vi "Down Sample Data.vi"(7 "Data log":enum16{"1 Hz", "10 Hz"}(ring), 8 "error in (no error)":errorcluster, 11 "location":path) -> (0 "error out":errorcluster)   [LabVIEW 2018]
uses:
  <vilib>/Analysis/baseanly.llb/Mean (DBL).vi
  <vilib>/Utility/file.llb/Read Delimited Spreadsheet (string).vi
  <vilib>/Utility/file.llb/Write Delimited Spreadsheet (string).vi
  <vilib>/Analysis/NI_AALBase.lvlib
panel:
  out "array type (2D Dbl)":string[][](array[string])
  out "output array":string[][](array[string])
  out "subarray":string[][](array[string])
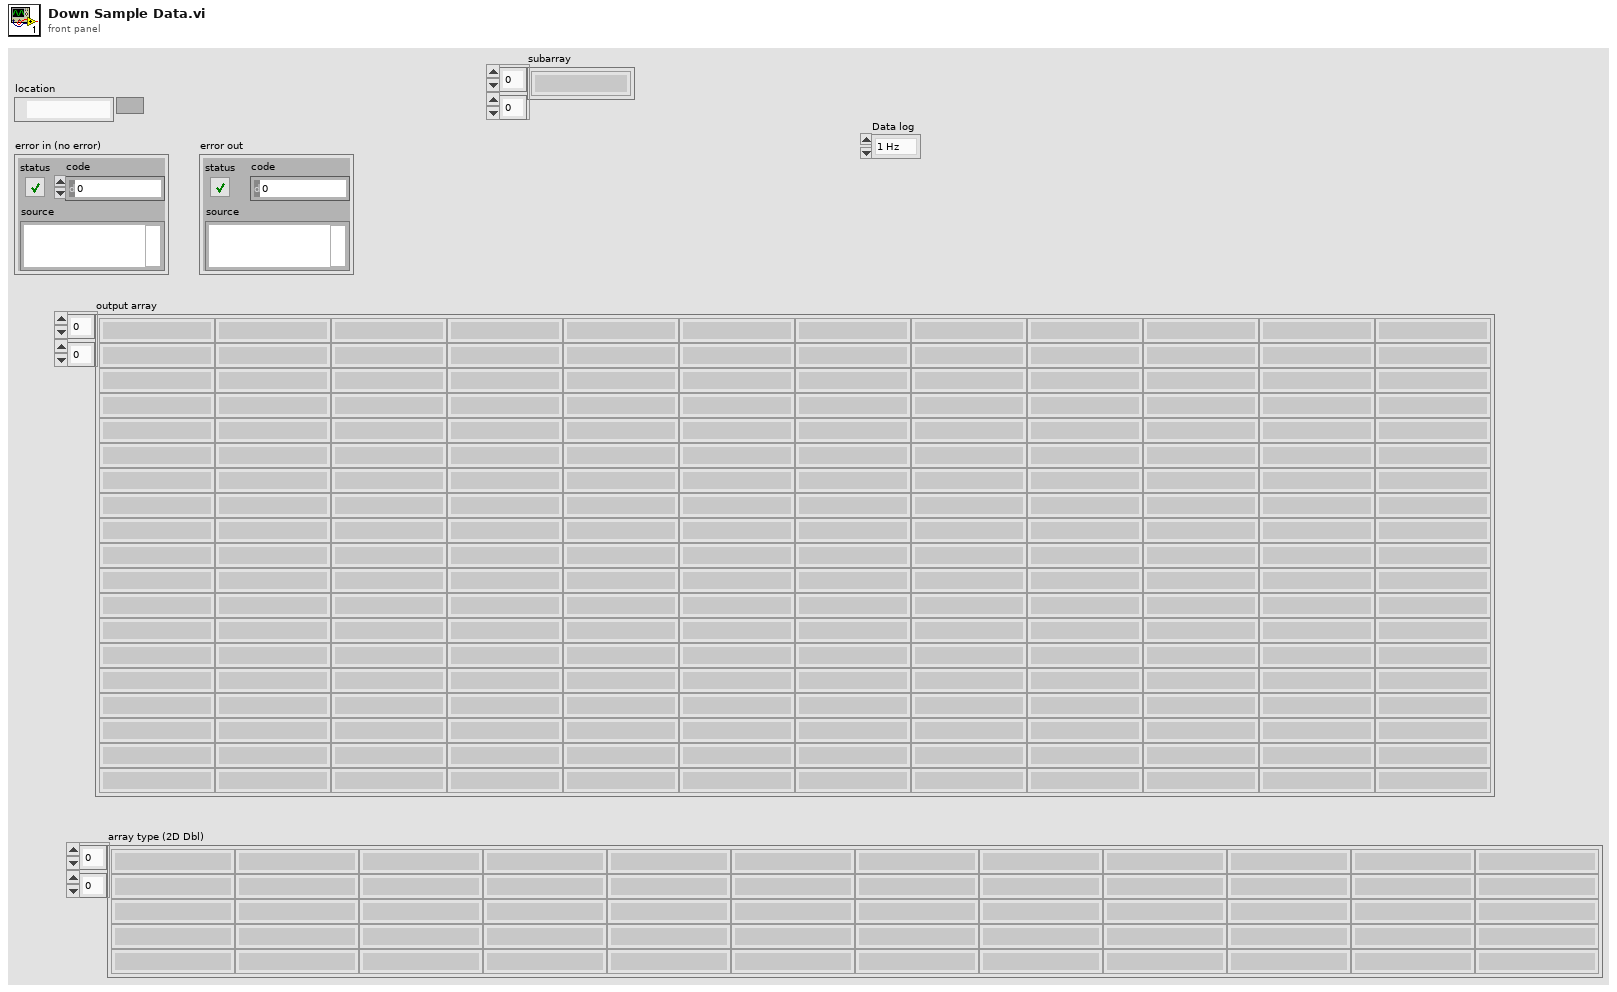
[diagram p1: front panel]
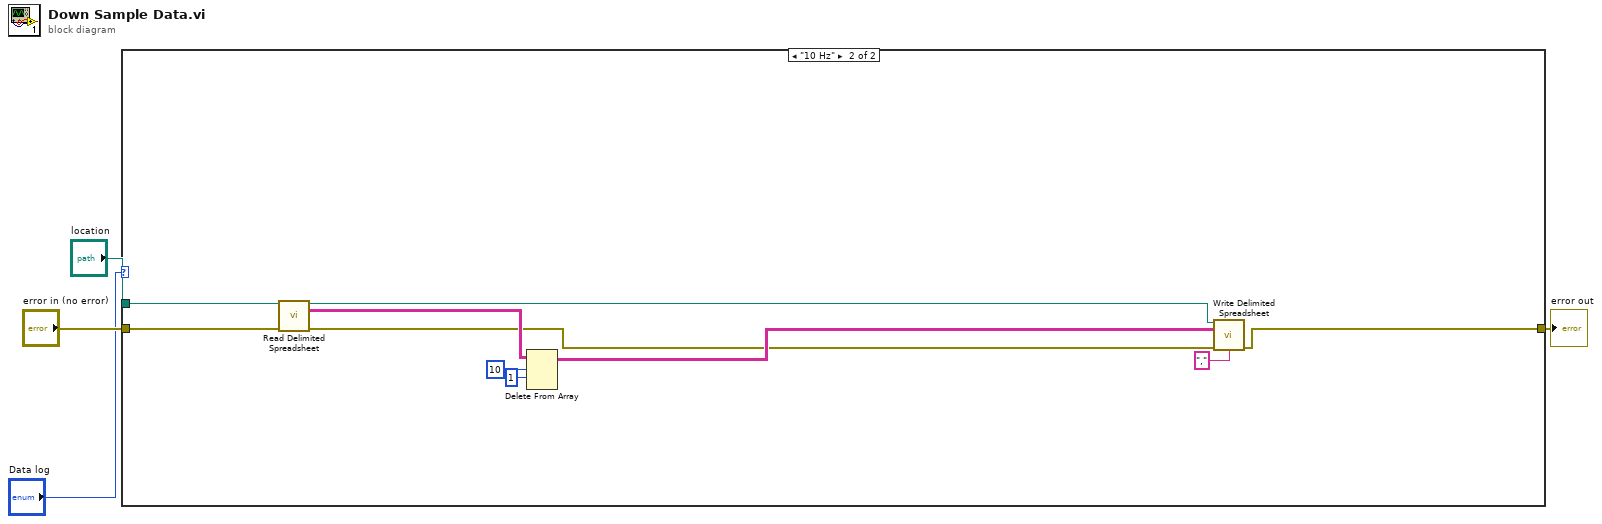
[diagram p0: block diagram]
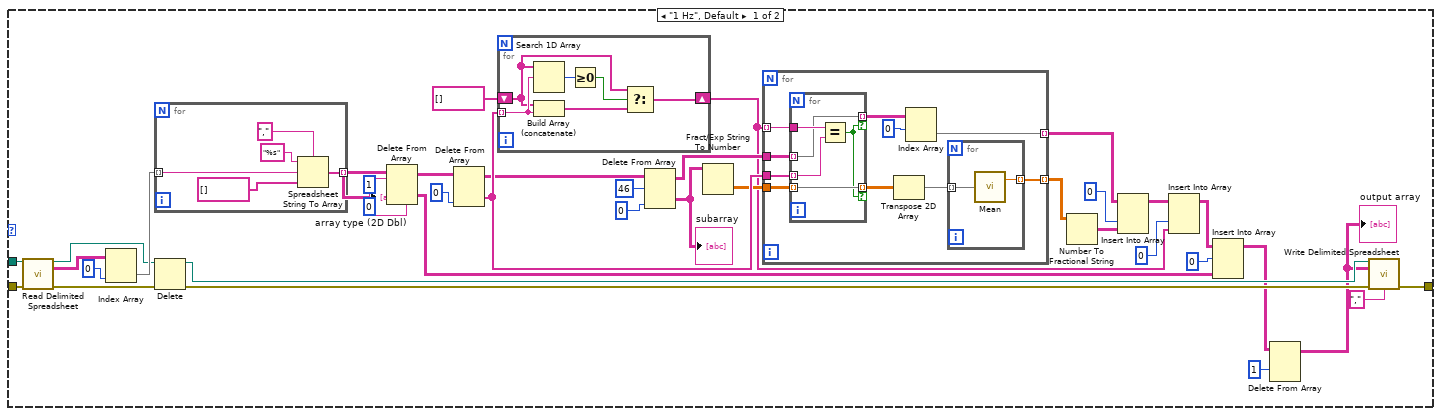
[diagram p2: hidden frame]
diagram:
  n1 = case shown="\"10 Hz\"" "Data log" {
    tunnel: "error in (no error)" -> [w35 w79]
    tunnel: "location" -> [w34 w78]
    tunnel: [w10 w70] -> w2
    frame "1 Hz", Default {
      n2 = call-poly <vilib>:"Read Delimited Spreadsheet.vi"("file path (dialog if empty)"=w34, "error in (no error)"=w35) -> ("new file path (Not A Path if cancelled)"=w13:path, "all rows"=w38:string[][], "error out"=w11:errorcluster)  [unwired: 8 in, 3 out]
      n3 = Index Array(array=w38, index (col)=0 ("disabled index (col)")) -> (element=w37:string[])  [unwired: 1 in]
      n4 = for {
        tunnel: w37 -> [w68] mode=indexing
        tunnel: [w65] -> w39 mode=indexing
        n5 = Spreadsheet String To Array(delimiter (Tab)=",", format string="%s", spreadsheet string=w68, array type (2D Dbl)=string[] []) -> (array=w65:string[])
      }
      "array type (2D Dbl)" <- w39
      n6 = Delete(path (use dialog)=w13, error in=w11) -> (deleted path=w12:path, error out=w9:errorcluster)  [unwired: 3 in, 1 out]
      n7 = Delete From Array(array=w39, length=1, index (row)=0 ("disabled index (row)")) -> (deleted portion=w15:string[][], array with subset deleted=w32:string[][])  [unwired: 1 in]
      n8 = Delete From Array(array=w32, index (col)=0 ("disabled index (col)")) -> (deleted portion=w30:string[], array with subset deleted=w26:string[][])  [unwired: 2 in]
      n9 = for {
        shift-right: [w59] -> w18
        shift-left: string[] [] ("array type (2D Dbl)") -> [w61]
        tunnel: w30 -> [w64] mode=indexing
        n10 = Search 1D Array(1D array=w61, element=w64) -> (index of element=w63:i32)  [unwired: 1 in]
        n11 = Build Array (concatenate)(w61, w64) -> (w60:string[])
        n12 = Greater Or Equal To 0?(x=w63) -> (x >= 0?=w62:bool)
        n13 = Select(t=w61, s=w62, f=w60) -> (s? t:f=w59:string[])
      }
      n14 = Delete From Array(array=w26, length=46, index (col)=0 ("disabled index (col)")) -> (deleted portion=w29:string[][], array with subset deleted=w24:string[][])  [unwired: 1 in]
      "subarray" <- w29
      n15 = Fract/Exp String To Number(string=w29) -> (number=w28:dbl[][])  [unwired: 3 in, 1 out]
      n16 = for {
        tunnel: w18 -> [w51] mode=indexing
        tunnel: w30 -> [w50]
        tunnel: w28 -> [w49]
        tunnel: [w46] -> w14 mode=indexing
        tunnel: w24 -> [w45]
        tunnel: [w42] -> w23 mode=indexing
        n17 = for {
          tunnel: w51 -> [w58]
          tunnel: w50 -> [w57] mode=indexing
          tunnel: w49 -> [w56] mode=indexing
          tunnel: [w56] -> w48 mode=indexing if=w54
          tunnel: w45 -> [w55] mode=indexing
          tunnel: [w55] -> w44 mode=indexing if=w54
          n18 = Equal?(x=w58, y=w57) -> (x = y?=w54:bool)
        }
        n19 = Transpose 2D Array(2D array=w48) -> (transposed array=w47:dbl[][])
        n20 = Index Array(array=w44, index (row)=0) -> (element=w42:string[])  [unwired: 1 in]
        n21 = for {
          tunnel: w47 -> [w53] mode=indexing
          tunnel: [w52] -> w46 mode=indexing
          n22 = call-poly <vilib>:"Mean.vi"("X"=w53) -> ("mean"=w52:dbl)  [unwired: 1 out]
        }
      }
      n23 = Number To Fractional String(number=w14) -> (F-format string=w22:string[][])  [unwired: 3 in]
      n24 = Insert Into Array(array=w23, index (col)=0 ("disabled index (col)"), new element=w22) -> (w20:string[][])  [unwired: 1 in]
      n25 = Insert Into Array(array=w20, index (col)=0 ("disabled index (col)"), new element=w18) -> (w17:string[][])  [unwired: 1 in]
      n26 = Insert Into Array(array=w17, index (row)=0, new element=w15) -> (w7:string[][])  [unwired: 1 in]
      n27 = Delete From Array(array=w7, index (row)=1) -> (array with subset deleted=w6:string[][])  [unwired: 2 in, 1 out]
      "output array" <- w6
      n28 = call-poly <vilib>:"Write Delimited Spreadsheet.vi"("file path (dialog if empty)"=w12, "2D data"=w6, "error in (no error)"=w9, "delimiter (\\t)"="," ("delimiter (\\t)")) -> ("error out"=w10:errorcluster)  [unwired: 10 in, 1 out]
    }
    frame "10 Hz" {
      n29 = call-poly <vilib>:"Read Delimited Spreadsheet.vi"("file path (dialog if empty)"=w78, "error in (no error)"=w79) -> ("new file path (Not A Path if cancelled)"=w72:path, "all rows"=w77:string[][], "error out"=w71:errorcluster)  [unwired: 8 in, 3 out]
      n30 = Delete From Array(array=w77, length=10, index (row)=1) -> (array with subset deleted=w73:string[][])  [unwired: 1 in, 1 out]
      n31 = call-poly <vilib>:"Write Delimited Spreadsheet.vi"("file path (dialog if empty)"=w72, "2D data"=w73, "error in (no error)"=w71, "delimiter (\\t)"="," ("delimiter (\\t)")) -> ("error out"=w70:errorcluster)  [unwired: 10 in, 1 out]
    }
  }
  "error out" <- w2
